vi "Display Input (DBL) Popup (GIF).vi"(4 "Message Size":T1={"Message Height"=-1, "Message Width"=-1, "Message Location"=enum."Bottom"} {"Message Width" min=-1 step=1; "Message Height" min=-1 step=1}, 6 "Theme":refnum<class "Theme.lvclass">, 8 "Error In":errorcluster, 9 "Default Input":dbl, 10 "Message":string, 11 "Graphic":path) -> (0 "Error Out":errorcluster, 1 "Input Value":dbl)   [LabVIEW 2021, in "GIF - Input (DBL).lvclass"]
doc: "The input (DBL) popup will display information to the user and wait for the operator to enter a value and click the button.\n\n<b>Note:</b> This popup type allows the user to define a custom image for the display. The developer should test all settings prior to deployment to make sure that all images and text fit on the screen correctly.\n\n<b>Note:</b> The function <b>Close Pop-Up (DBL).vi</b> can be used to send a value when closing this dialog. Otherwise, use Close Pop-Up.vi to close it early.\n\nInputs:\n-Graphic [path] - path to the image file to display\n-Message [String] - String Variable to populate Display with\n-Theme [lvclass] - the theme class for the pop up\n-Default Input [DBL] - default value for the prompt\n\nOutputs\n-InputValue [DBL] - the user's input data\n\n<b>Code Developed By:</b>\nDaniel Coons\nTechnology Service Corporation\n1983 S Liberty Drive\nBloomington, IN 47403\nPhone: 812 558-7100\ndaniel.coons@tsc.com\nwww.tsc.com/atcs"
uses:
  GIF - Input (DBL).lvclass
  <vilib>/addons/_TSC/TSC Pop-Up/Theme/Theme.lvclass
  <vilib>/addons/_TSC/TSC Pop-Up/Popup/message info--typedef.ctl
  GIF - Input (DBL).lvclass/GIF - Input (DBL).ctl
  <vilib>/addons/_TSC/TSC Pop-Up/Popup/Popup.lvclass
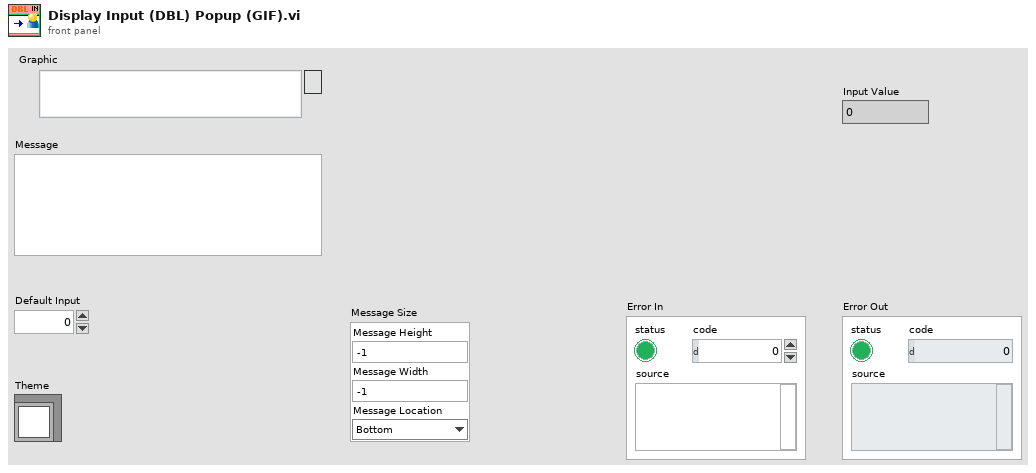
[diagram p1: front panel]
types:
  T1 = typedef "Pop-Up.lvlib/Popup.lvclass/message info--typedef.ctl" = cluster{"Message Height":i32, "Message Width":i32, "Message Location":enum16{"Top", "Bottom", "Right", "Left"}}
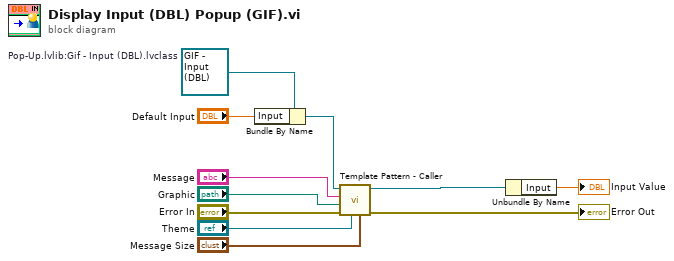
[diagram p0: block diagram]
diagram:
  w1 = refnum<class "GIF - Input (DBL).lvclass"> refnum  # Pop-Up.lvlib:Gif - Input (DBL).lvclass
  n1 = Bundle By Name(cluster=w1, "Input"="Default Input") -> (w5:refnum<class "GIF - Input (DBL).lvclass">)
  n2 = call-dynamic "Template Pattern - Caller.vi"("Message Size"="Message Size", "Theme"="Theme", "error in (no error)"="Error In", "Graphic"="Graphic", "Message"="Message", "Pop-Up in"=w5) -> ("error out"=→"Error Out":errorcluster, "Pop-Up out"=w8:refnum<class "GIF - Input (DBL).lvclass">)  [unwired: 4 in]
  n3 = Unbundle By Name(w8) -> ("Input"=→"Input Value":dbl)
